vi "Create Board.vi"(8 "error in (no error)":errorcluster, 10 "Board Size":u16, 11 "Board in":refnum<class "Board.lvclass">) -> (0 "error out":errorcluster, 3 "Board out":refnum<class "Board.lvclass">)   [LabVIEW 2017, in "Board.lvclass"]
uses:
  Board.lvclass
  Board.lvclass/Board.ctl
  <vilib>/LIEF/Forms/Shape/Shape.lvclass
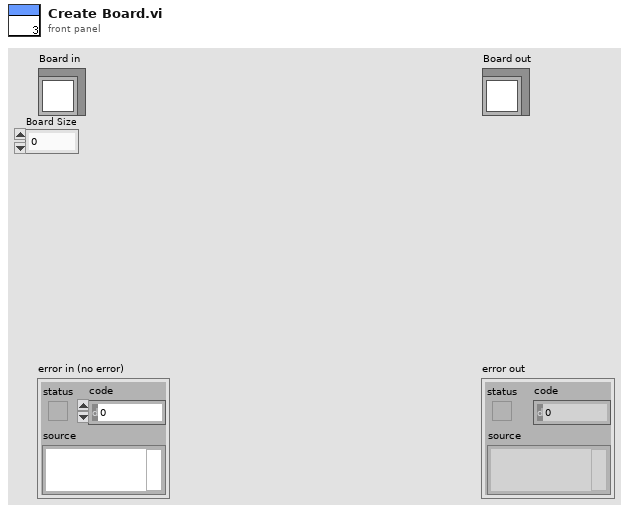
[diagram p1: front panel]
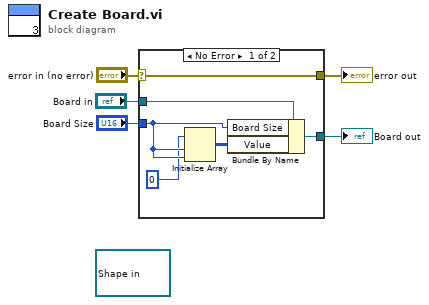
[diagram p0: block diagram]
diagram:
  (unwired) refnum<data-value> refnum ("New Block")
  n1 = case shown="No Error" "error in (no error)" {
    selector: "error in (no error)" -> [w11 w13]
    tunnel: [w11 w13] -> w4
    tunnel: [w9 w12] -> w2
    tunnel: "Board in" -> [w10 w12]
    tunnel: "Board Size" -> [w8 _]
    frame No Error {
      n2 = Initialize Array(u32 0, w8, w8) -> (w6:u32[][])
      n3 = Bundle By Name(cluster=w10, "Board Size"=w8, "Value"=w6) -> (w9:refnum<class "Board.lvclass">)
    }
    frame Error {
    }
  }
  "error out" <- w4
  "Board out" <- w2
